vi "test8-LocalExternalStateRegistration.vi"(8 "error in (no error)":errorcluster, 11 "TestCase in":refnum<class "testcase-CSMBroadcast.lvclass">) -> (0 "error out":errorcluster, 3 "TestCase out":refnum<class "testcase-CSMBroadcast.lvclass">)   [LabVIEW 2017, in "testcase-CSMBroadcast.lvclass"]
uses:
  testcase-CSMBroadcast.lvclass
  0b17d103-e67b-41be-a9eb-a2ee1311ff1f.vi
  5999693e-4f8a-4b34-ae87-f34dff5771be.vi
  52a2a10a-a04b-4bad-8df4-e1eb944f47cc.vi
  826f03dd-b4b5-4c6b-9085-8edf6da4f43b.vi
  src/user.lib/_NEVSTOP/Communicable State Machine(CSM)/AdvanceAPI/CSM - Revert Arguments-Safe String.vi
  src/user.lib/_NEVSTOP/Communicable State Machine(CSM)/_Shared/Trim Single-line Text.vi
  src/user.lib/_NEVSTOP/Communicable State Machine(CSM)/AdvanceAPI/CSM - Make String Arguments Safe.vi
  src/user.lib/_NEVSTOP/Communicable State Machine(CSM)/AdvanceAPI/CSM - Break Down Multiple States String.vi
  src/user.lib/_NEVSTOP/Communicable State Machine(CSM)/AdvanceAPI/CSM - Keywords.vi
  src/user.lib/_NEVSTOP/Communicable State Machine(CSM)/_Polymophic/CSM - Replace Marks in Messages.vi
  src/user.lib/_NEVSTOP/Communicable State Machine(CSM)/AdvanceAPI/CSM - Get Module Attribute.vi
  <vilib>/addons/_JKI Toolkits/VI Tester/TestCase.llb/TestCase.lvclass
  src/user.lib/_NEVSTOP/Communicable State Machine(CSM)/Communicable State Machine.lvlib
  C:/Program Files (x86)/National Instruments/LabVIEW 2017/vi.lib/addons/_JKI Toolkits/VI Tester/TestCase.llb/TestCase.lvclass
panel:
  out "One-Shot Unregistrations":string
  out "One-Shot Registrations":string
  out "LoopCount 2":i32
  out "State History":string
  out "LoopCount":i32
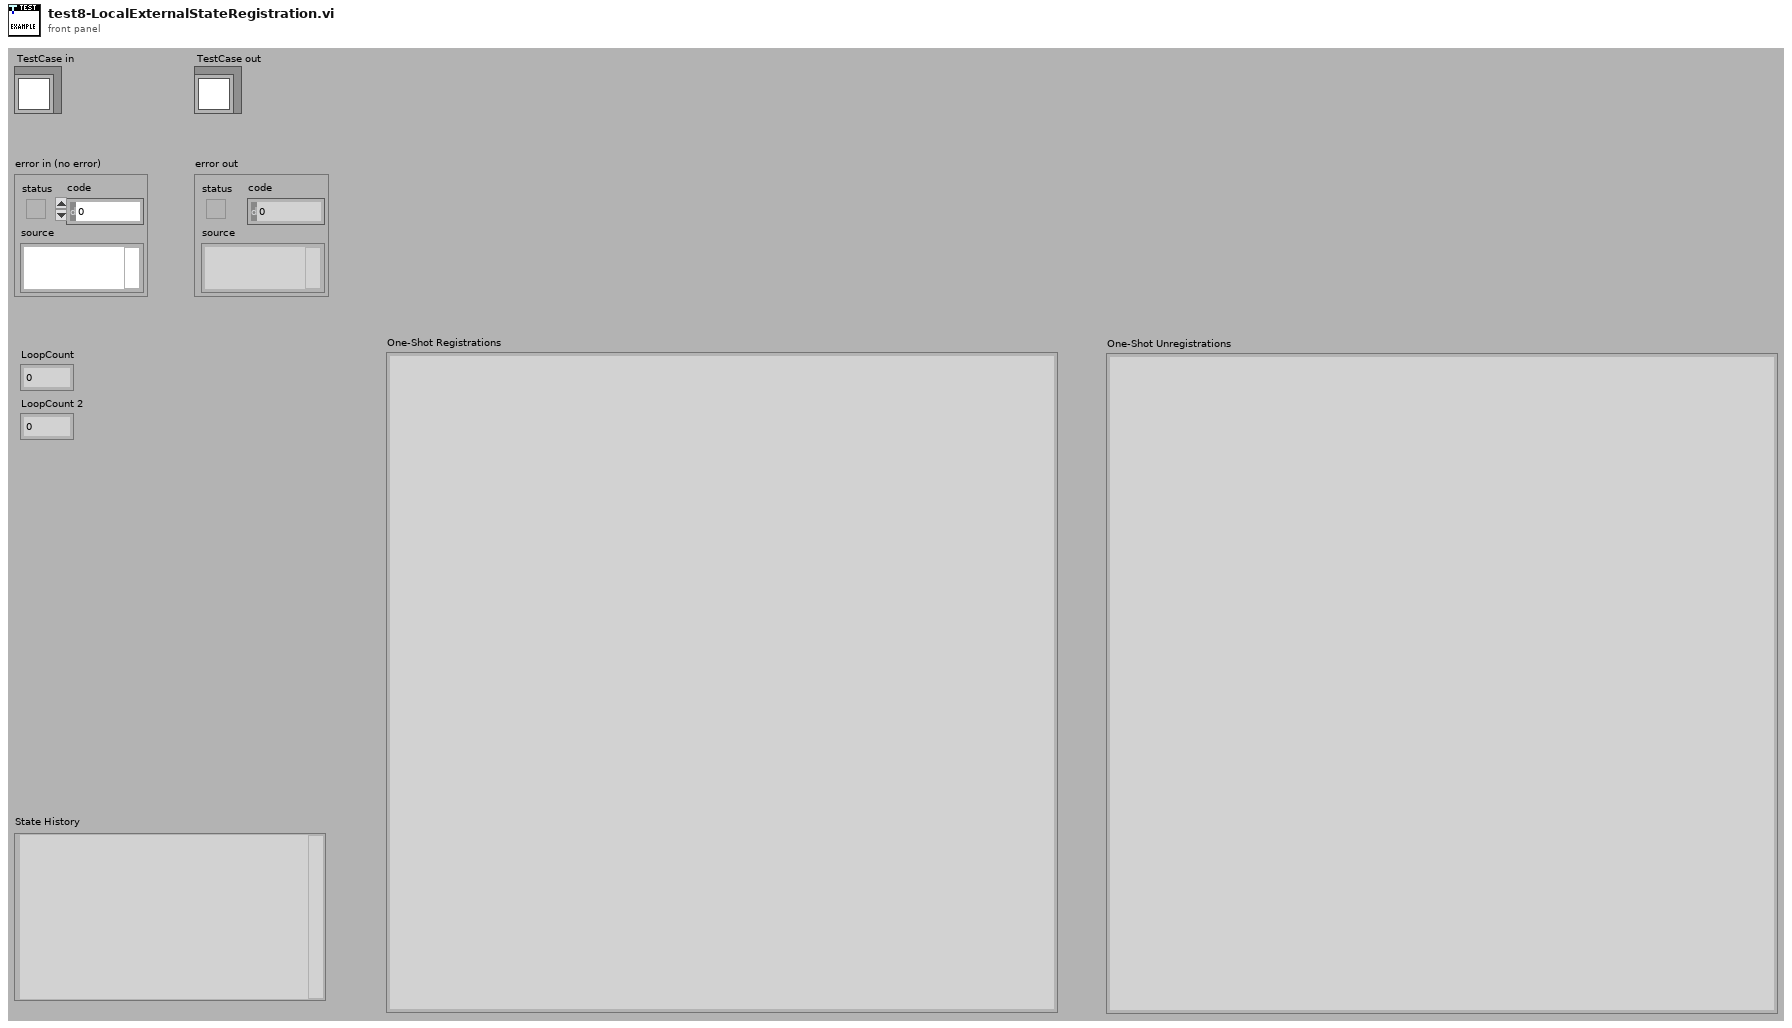
[diagram p1: front panel]
types:
  T1 = enum32{"Invalid", "Standard", "Closed", "Hidden", "Minimized", "Maximized"}
  T2 = enum32{"invalid app kind", "Development System", "Run Time System", "Student Edition", "Embedded LabVIEW", "Evaluation", "Custom"}
  T3 = typedef "Communicable State Machine.lvlib/_CSM_Response Source Message.ctl" = cluster{"‘State":string, "’Arguments":string, "’Error":errorcluster}
  T4 = cluster{"Current VI Reference":refnum<vi>, "Close Panel on Exit?":bool}
  T5 = cluster{"Core":cluster{"Current VI Reference":refnum<vi>, "Close Panel on Exit?":bool}, "Your Boolean data":bool, "Your string data":string}
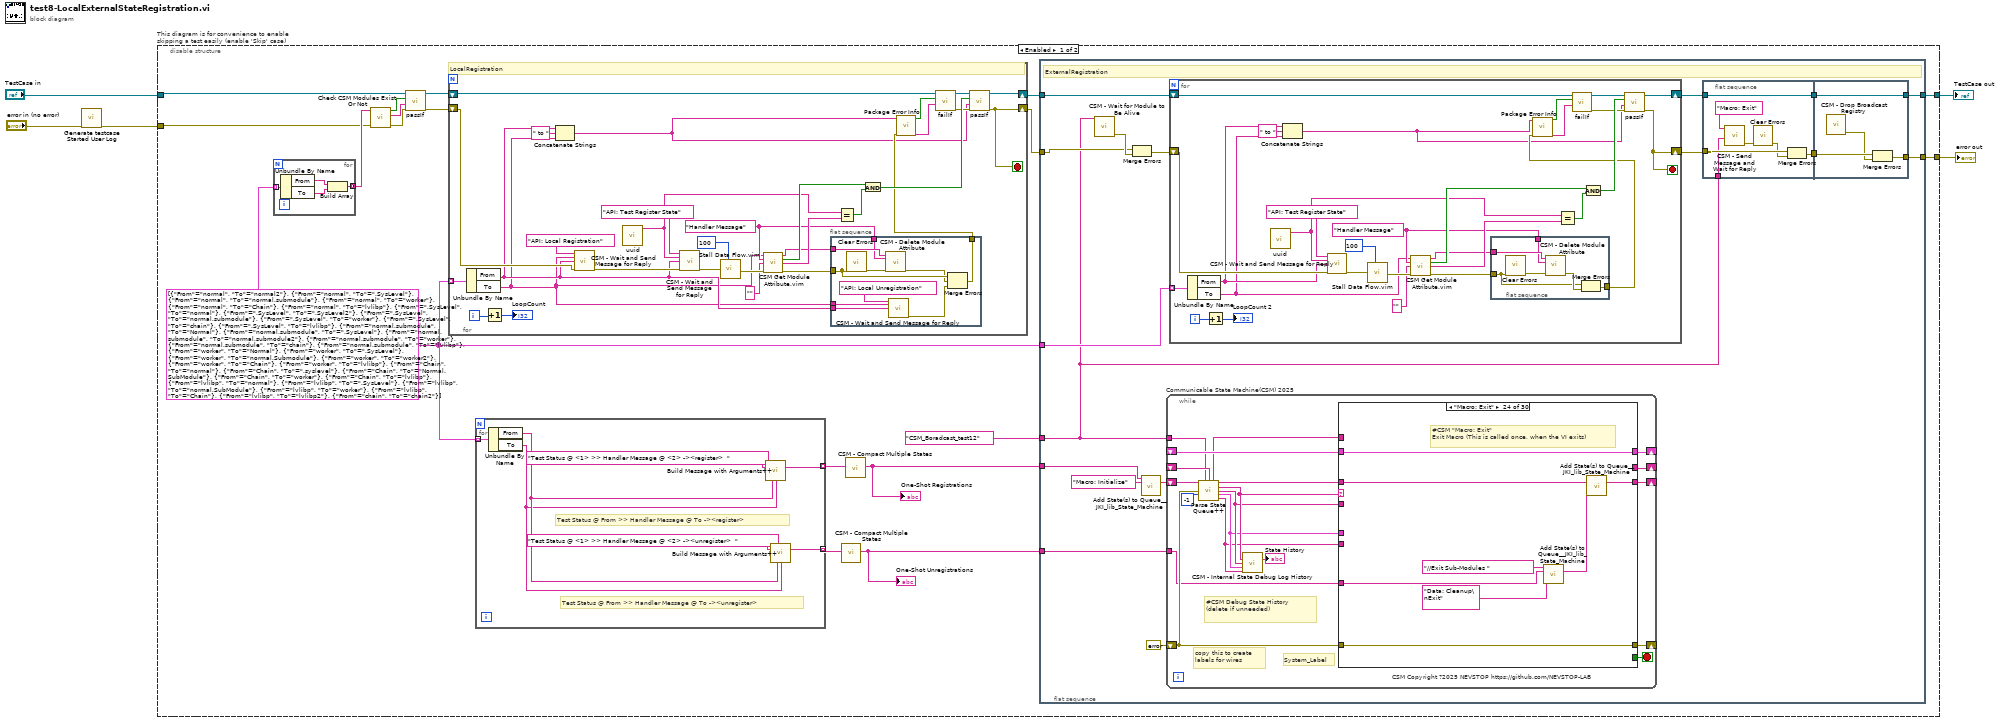
[diagram p0: block diagram]
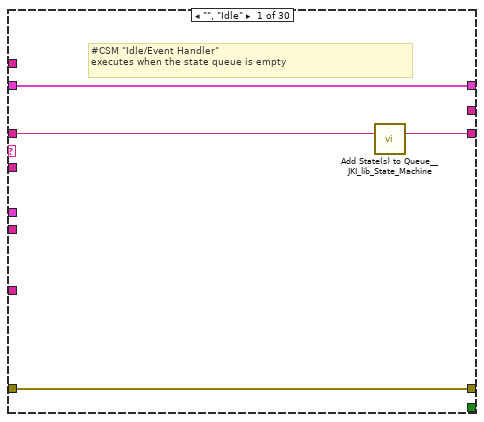
[diagram p2: hidden frame]
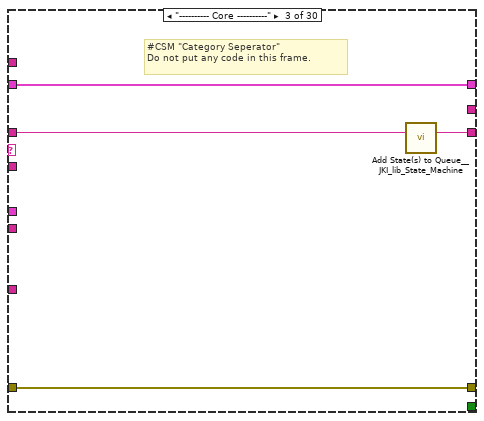
[diagram p4: hidden frame]
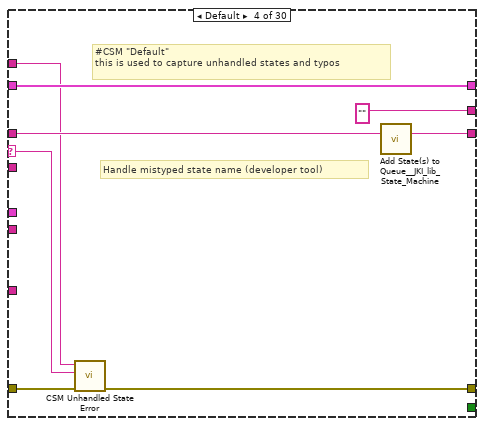
[diagram p5: hidden frame]
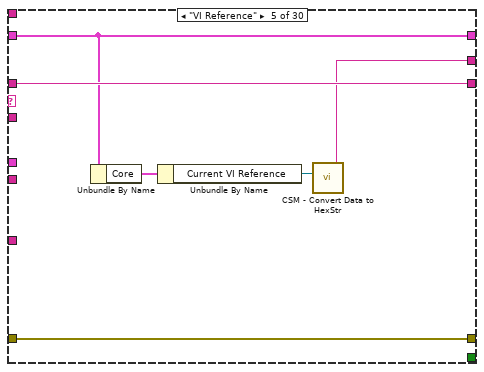
[diagram p6: hidden frame]
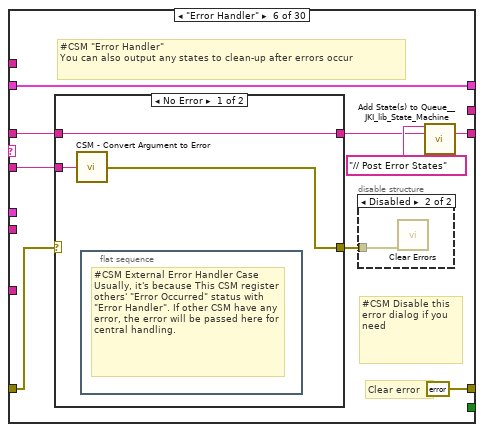
[diagram p7: hidden frame]
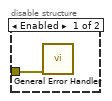
[diagram p8: hidden frame]
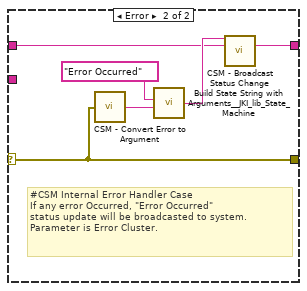
[diagram p9: hidden frame]
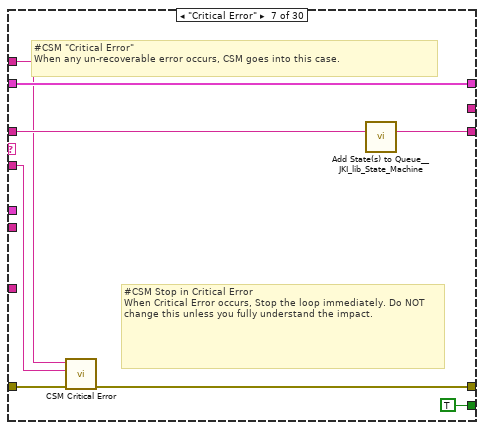
[diagram p10: hidden frame]
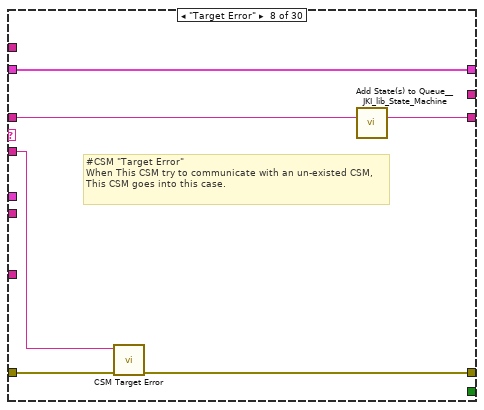
[diagram p11: hidden frame]
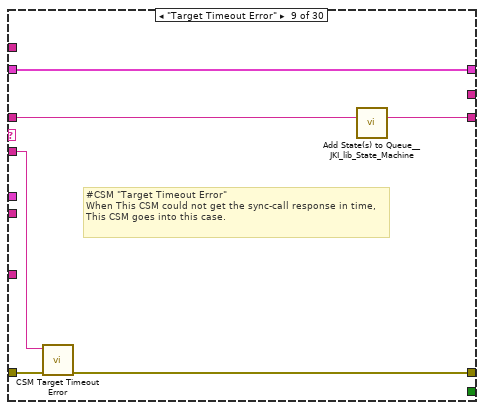
[diagram p12: hidden frame]
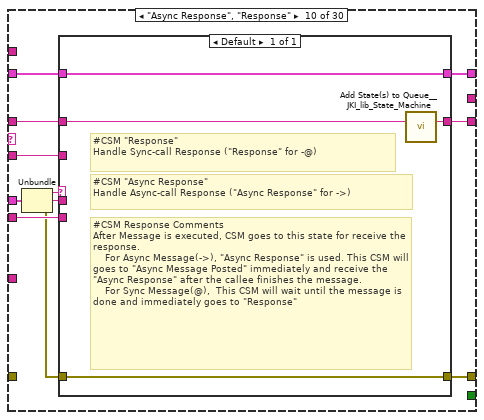
[diagram p13: hidden frame]
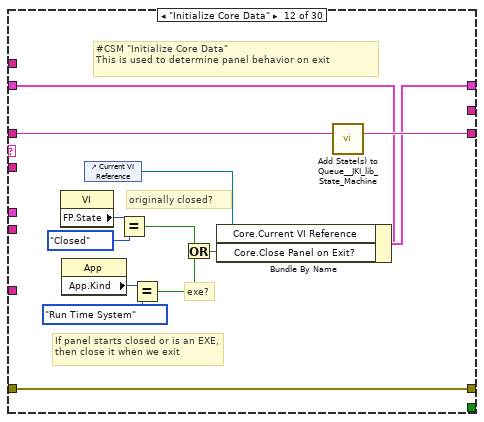
[diagram p15: hidden frame]
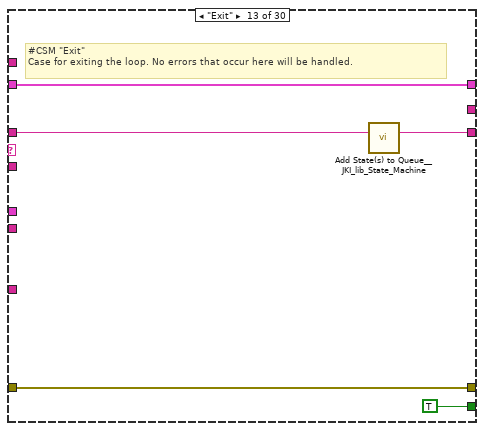
[diagram p16: hidden frame]
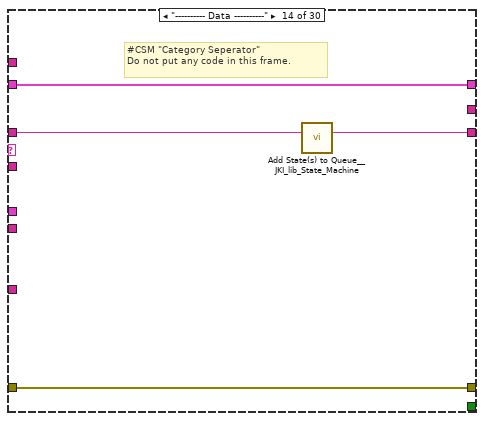
[diagram p17: hidden frame]
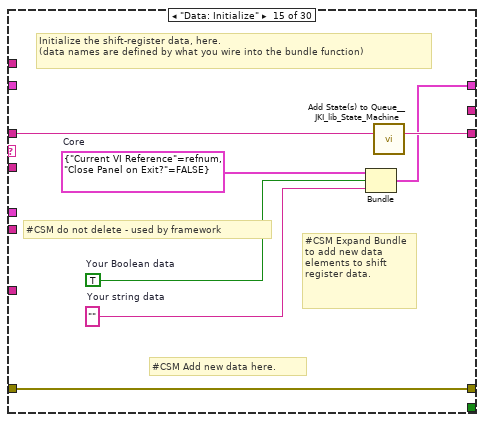
[diagram p18: hidden frame]
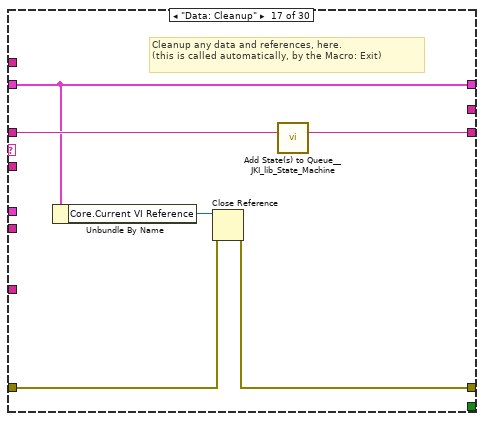
[diagram p20: hidden frame]
diagram:
  n1 = call "Generate testcase Started User Log.vi"("Error In"="error in (no error)") -> ("error out"=w1:errorcluster)  [unwired: 10 in]
  n2 = disable-structure "This diagram is for convenience to enable skipping a test easily (enable 'Skip' case)" shown="Enabled" {
    disable-tunnel: "TestCase in" -> [w11 w419]
    disable-tunnel: [w7 w417] -> w2
    disable-tunnel: [w17 w418] -> w4
    disable-tunnel: w1 -> [w8 w416]
    frame Enabled {
      w12 = cluster{"From":string, "To":string}[] [{"From"="normal", "To"="normal2"}, {"From"="normal", "To"=".SysLevel"}, {"From"="normal", "To"="normal.submodule"}, {"From"="normal", "To"="worker"}, {"From"="normal", "To"="Chain"}, {"From"="normal", "To"="lvlibp"}, {"From"=".SysLevel", "To"="normal"}, {"From"=".SysLevel", "To"=".SysLevel2"}, {"From"=".SysLevel", "To"="normal.submodule"}, {"From"=".SysLevel", "To"="worker"}, {"From"=".SysLevel", "To"="chain"}, {"From"=".SysLevel", "To"="lvlibp"}, {"From"="normal.submodule", "To"="Normal"}, {"From"="normal.submodule", "To"=".SysLevel"}, {"From"="normal.submodule", "To"="normal.submodule2"}, {"From"="normal.submodule", "To"="worker"}, {"From"="normal.submodule", "To"="chain"}, {"From"="normal.submodule", "To"="lvlibp"}, {"From"="worker", "To"="Normal"}, {"From"="worker", "To"=".SysLevel"}, {"From"="worker", "To"="normal.Submodule"}, {"From"="worker", "To"="worker2"}, {"From"="worker", "To"="Chain"}, {"From"="worker", "To"="lvlibp"}, {"From"="Chain", "To"="normal"}, {"From"="Chain", "To"=".syslevel"}, {"From"="Chain", "To"="Normal.SubModule"}, {"From"="Chain", "To"="worker"}, {"From"="Chain", "To"="lvlibp"}, {"From"="lvlibp", "To"="normal"}, {"From"="lvlibp", "To"=".SysLevel"}, {"From"="lvlibp", "To"="normal.SubModule"}, {"From"="lvlibp", "To"="worker"}, {"From"="lvlibp", "To"="Chain"}, {"From"="lvlibp", "To"="lvlibp2"}, {"From"="chain", "To"="chain2"}]
      n3 = for {
        tunnel: w12 -> [w27] mode=indexing
        tunnel: [w24] -> w15 mode=concatenating
        n4 = Unbundle By Name(w27) -> ("From"=w26:string, "To"=w25:string)
        n5 = Build Array(w26, w25) -> (w24:string[])
      }
      n6 = call "Check CSM Modules Exist Or Not.vi"("error in"=w8, "CSM names in"=w15) -> ("error out"=w13:errorcluster, "Debug string"=w14:string, "All Modules Exist?"=w16:bool)  [unwired: 7 in]
      n7 = call-dynamic "passIf.vi"("error in (no error)"=w13, "message (\"\")"=w14, "pass"=w16, "TestCase in"=w11) -> ("error out"=w9:errorcluster, "TestCase out"=w10:refnum<class "testcase-CSMBroadcast.lvclass">)  [unwired: 6 in]
      n8 = for {
        shift-right: [w38] -> w22
        shift-left: w9 -> [w39]
        shift-right: [w45] -> w23
        shift-left: w10 -> [w35]
        tunnel: w12 -> [w56] mode=indexing
        i -> [w58]
        stop <- w38 stop-if-true
        w40 = "Handler Message" ("To")
        # "LocalRegistration"
        n9 = Unbundle By Name(w56) -> ("From"=w31:string, "To"=w30:string)
        n10 = Increment(x=w58) -> (x+1=→"LoopCount":i32)
        n11 = Concatenate Strings(w31, " to " ("string"), w30) -> (w28:string)
        n12 = call "CSM - Wait and Send Message for Reply.vi"("State"="API: Local Registration", "Arguments (\"\")"=w30, "Target Module"=w31, "Error In (No Error)"=w39) -> ("error out"=w53:errorcluster)  [unwired: 8 in, 3 out]
        n13 = call "uuid.vi"() -> ("UUID"=w47:string)  [unwired: 11 in]
        n14 = call "CSM - Wait and Send Message for Reply.vi"("State"="API: Test Register State", "Arguments (\"\")"=w47, "Target Module"=w31, "Error In (No Error)"=w53) -> ("error out"=w52:errorcluster)  [unwired: 8 in, 3 out]
        n15 = call "Stall Data Flow.vim"("value in"=w52, "milliseconds to wait"=u32 100) -> ("value out"=w50:errorcluster)  [unwired: 1 out]
        n16 = call "CSM Get Module Attribute.vim"("CSM Name"=w30, "Attribute"=w40, "Default Value (Empty Variant)"="", "Error In"=w50) -> ("CSM Name (Dup)"=w41:string, "Found"=w49:bool, "Value"=w46:string, "error out"=w42:errorcluster)  [unwired: 7 in, 1 out]
        n17 = flat-sequence {
          tunnel: w42 -> [w62]
          tunnel: w41 -> [w67]
          tunnel: w40 -> [w66]
          tunnel: w30 -> [w64]
          tunnel: w31 -> [w63]
          tunnel: [w59] -> w32
          frame #0 {
            n18 = call <vilib>:"Clear Errors.vi"("error in (no error)"=w62) -> ("error out"=w68:errorcluster)  [unwired: 5 in, 1 out]
            n19 = call "CSM - Delete Module Attribute.vi"("CSM Name"=w67, "Attribute"=w66, "Error In"=w68) -> ("error out"=w61:errorcluster)  [unwired: 9 in, 3 out]
            n20 = call "CSM - Wait and Send Message for Reply.vi"("State"="API: Local Unregistration", "Arguments (\"\")"=w64, "Target Module"=w63) -> ("error out"=w60:errorcluster)  [unwired: 9 in, 3 out]
            n21 = Merge Errors(w62, w61, w60) -> (w59:errorcluster)
          }
        }
        n22 = Equal?(x=w47, y=w46) -> (x = y?=w44:bool)
        n23 = And(x=w49, y=w44) -> (x .and. y?=w43:bool)
        n24 = call "Package Error Info.vi"("error in"=w32, "String in"=w28) -> ("packed error info out"=w36:string, "error status"=w37:bool)  [unwired: 8 in]
        n25 = call-dynamic "failIf.vi"("message (\"\")"=w36, "fail"=w37, "TestCase in"=w35) -> ("error out"=w33:errorcluster, "TestCase out"=w34:refnum<class "testcase-CSMBroadcast.lvclass">)  [unwired: 7 in]
        n26 = call-dynamic "passIf.vi"("error in (no error)"=w33, "message (\"\")"=w28, "pass"=w43, "TestCase in"=w34) -> ("error out"=w38:errorcluster, "TestCase out"=w45:refnum<class "testcase-CSMBroadcast.lvclass">)  [unwired: 6 in]
      }
      n27 = for {
        tunnel: w12 -> [w74] mode=indexing
        tunnel: [w73] -> w21 mode=indexing
        tunnel: [w69] -> w19 mode=indexing
        # "Test Status @ From >> Handler Message @ To -><unregister>"
        # "Test Status @ From >> Handler Message @ To -><register>"
        n28 = Unbundle By Name(w74) -> ("From"=w71:string, "To"=w70:string)
        n29 = call-poly "Build Message with Arguments++.vi"("States With Replace Token"="Test Status @ <1> >> Handler Message @ <2> -><register>  " ("State"), "<1>"=w71, "<2>"=w70) -> ("States"=w73:string)  [unwired: 12 in]
        n30 = call-poly "Build Message with Arguments++.vi"("States With Replace Token"="Test Status @ <1> >> Handler Message @ <2> -><unregister>  " ("State"), "<1>"=w71, "<2>"=w70) -> ("States"=w69:string)  [unwired: 12 in]
      }
      n31 = call "CSM - Compact Multiple States.vi"("Multiple States"=w19) -> ("States"=w18:string)  [unwired: 9 in]
      "One-Shot Unregistrations" <- w18
      n32 = call "CSM - Compact Multiple States.vi"("Multiple States"=w21) -> ("States"=w20:string)  [unwired: 9 in]
      "One-Shot Registrations" <- w20
      n33 = flat-sequence {
        tunnel: w23 -> [w89]
        tunnel: w22 -> [w83]
        tunnel: w12 -> [w88]
        tunnel: w20 -> [w86]
        tunnel: w18 -> [w82]
        tunnel: [w80] -> w17
        tunnel: [w77] -> w7
        tunnel: "CSM_Boradcast_test12" ("Name (\"\" to Use UUID)") -> [w76]
        frame #0 {
          # "ExternalRegistration"
          n34 = call "CSM - Wait for Module to Be Alive.vi"("CSM Name"=w76) -> ("error out"=w87:errorcluster)  [unwired: 12 in, 2 out]
          n35 = Merge Errors(w83, w87) -> (w84:errorcluster)
          n36 = call <vilib>:"Add State(s) to Queue__JKI_lib_State_Machine.vi"("State(s) in Front (\"\")"=w86, "State(s) in (\"\")"="Macro: Initialize" ("Init State(\"Macro: Initialize\")")) -> ("States Out"=w90:string)  [unwired: 13 in]
          n37 = while "Communicable State Machine(CSM) 2025" {
            shift-right: [w152] -> _
            shift-left: _ -> [w151]
            shift-right: [w155] -> _
            shift-left: errorcluster {"status"=FALSE, "code"=0, "source"=""} ("error out") -> [w150]
            shift-right: [w154] -> _
            shift-left: w90 -> [w156]
            shift-right: [w149] -> _
            shift-left: _ -> [w143]
            tunnel: w82 -> [w140]
            tunnel: w76 -> [w139]
            stop <- w153 stop-if-true
            # "#CSM Debug State History\n(delete if unneeded)"
            # "copy this to create labels for wires"
            # "System_Label"
            # "CSM Copyright ?2025 NEVSTOP https://github.com/NEVSTOP-LAB"
            n38 = call "Parse State Queue++.vi"("State Queue"=w156, "Name (\"\" to Use UUID)"=w139, "Response Arguments"=w143, "Previous Error"=w150, "Dequeue (1 ms)"=-1 ("Timeout")) -> ("Name Used"=w144:string, "Remaining States"=w157:string, "Current State"=w148:string, "Arguments"=w147:string, "Additional Information"=w146:T3, "Source CSM"=w145:string)  [unwired: 5 in]
            n39 = call "CSM - Internal State Debug Log History.vi"("State"=w148, "Arguments (\"\")"=w147, ">> Response Source Message >>"=w146, "Source (\"\")"=w145) -> ("Debug Log"=→"State History":string)  [unwired: 11 in]
            n40 = case shown="\"Macro: Exit\"" w148 {
              selector: w148 -> [_ _ _ w171 _ _ _ _ _ _ _ _ _ _ _ _ _ _ _ _ _ _ _ _ _ _ _ _ _ _]
              tunnel: w157 -> [w158 w163 w168 w175 w181 w187 w208 w214 w220 w228 w239 w253 w258 w262 w269 w271 w278 w282 w286 w292 w307 w376 w381 w389 w391 w395 w400 w407 w411 w415]
              tunnel: w147 -> [_ _ _ _ _ w186 w204 w213 w218 w227 _ _ _ _ _ _ _ _ _ w287 w301 _ _ _ _ _ w398 _ _ _]
              tunnel: w151 -> [w159 w162 w165 w173 w180 w190 w209 w215 w221 w230 w238 w246 w256 w259 _ w270 w273 w279 w284 w290 w303 w373 w378 w386 w390 w394 w399 w404 w408 w412]
              tunnel: [w160 w164 w166 w169 w182 errorcluster {"status"=FALSE, "code"=0, "source"=""} ("error out") w205 w211 w217 w233 w240 w250 w255 w260 w266 w272 w274 w280 w283 w288 w304 w374 w379 w387 w392 w396 w401 w405 w409 w413] -> w155
              tunnel: w150 -> [w160 w164 w166 w176 w182 w188 w210 w212 w219 _ w240 w250 w255 w260 w266 w272 w275 w280 w283 w289 w305 w374 w379 w387 w392 w396 w401 w405 w409 w413]
              tunnel: [w161 w163 w167 w174 w181 w183 w207 w216 w222 w229 w239 w252 w257 w261 w268 w271 w277 w281 w285 w291 w306 w375 w380 w388 w391 w395 w400 w406 w410 w414] -> w154
              tunnel: [_ _ _ _ _ _ TRUE _ _ _ _ _ TRUE _ _ _ _ _ _ _ _ _ _ _ _ _ _ _ _ _] -> w153
              tunnel: [w159 w162 w165 w173 w180 w190 w209 w215 w221 w231 w238 w251 w256 w259 w267 w270 w273 w279 w284 w290 w303 w373 w378 w386 w390 w394 w399 w404 w408 w412] -> w152
              tunnel: w145 -> [_ _ _ _ _ _ _ _ _ w225 _ _ _ _ _ _ _ _ _ _ _ _ _ _ _ _ _ _ _ _]
              tunnel: w146 -> [_ _ _ _ _ _ _ _ _ w232 _ _ _ _ _ _ _ _ _ _ _ _ _ _ _ _ _ _ _ _]
              tunnel: [_ _ _ "" w177 _ _ _ _ _ _ _ _ _ _ _ _ _ _ _ _ _ _ _ _ "API1 Response" w397 _ _ _] -> w149
              tunnel: w144 -> [_ _ _ w170 _ _ w203 _ _ _ _ _ _ _ _ _ _ _ _ _ _ _ _ _ _ _ _ _ _ _]
              tunnel: w140 -> [_ _ _ _ _ _ _ _ _ _ _ _ _ _ _ _ _ _ _ _ _ _ _ w382 _ _ _ _ _ _]
              frame "", "Idle" {
                # "#CSM \"Idle/Event Handler\"\nexecutes when the state queue is empty"
                n41 = call <vilib>:"Add State(s) to Queue__JKI_lib_State_Machine.vi"("State(s) in (\"\")"=w158) -> ("States Out"=w161:string)  [unwired: 14 in]
              }
              frame "CSM Documentation" {
                # "#CSM README FIRST\n\nCommunicable State Machine(CSM) is a LabVIEW application framework that builds upon JKI State Machine(JKISM). It follows the pattern of JKISM and extends the keywords to describe message communication between modules, including concepts such as Sync-Message, Async-Message, Subscription/Unsubscription of status - essential elements for creating reusable code modules. For more information, please visit the CSM wiki: https://nevstop-lab.github.io/CSM-Wiki/\n\nFor instructions on JKI State Machine, visit: http://jki.net/state-machine/\nFor information about CSM, visit: https://github.com/NEVSTOP-LAB"
                # "#CSM \"Documentation\"\nCase for holding CSM Documenation"
              }
              frame "---------- Core ----------" {
                # "#CSM \"Category Seperator\"\nDo not put any code in this frame."
                n42 = call <vilib>:"Add State(s) to Queue__JKI_lib_State_Machine.vi"("State(s) in (\"\")"=w168) -> ("States Out"=w167:string)  [unwired: 14 in]
              }
              frame Default {
                # "#CSM \"Default\"\nthis is used to capture unhandled states and typos"
                # "Handle mistyped state name (developer tool)"
                n43 = call "CSM Unhandled State Error.vi"("error in (no error)"=w176, "Undefined State"=w171, "CSM Name"=w170) -> ("error out"=w169:errorcluster)  [unwired: 8 in]
                n44 = call <vilib>:"Add State(s) to Queue__JKI_lib_State_Machine.vi"("State(s) in (\"\")"=w175) -> ("States Out"=w174:string)  [unwired: 14 in]
              }
              frame "VI Reference" {
                n45 = Unbundle By Name(w180) -> ("Core"=w179:T4)
                n46 = Unbundle By Name(w179) -> ("Current VI Reference"=w178:refnum<vi>)
                n47 = call "CSM - Convert Data to HexStr.vi"("Variant"=w178) -> ("HEX String (0-9,A-F)"=w177:string)  [unwired: 8 in]
              }
              frame "Error Handler" {
                # "#CSM Disable this error dialog if you need"
                # "#CSM \"Error Handler\"\nYou can also output any states to clean-up after errors occur"
                # "Clear error"
                n48 = case shown="No Error" w188 {
                  selector: w188 -> [_ w197]
                  tunnel: [w196 w199] -> w184
                  tunnel: w187 -> [w196 w198]
                  tunnel: w186 -> [w195 _]
                  tunnel: [w194 w197] -> w189
                  frame No Error {
                    n49 = call "CSM - Convert Argument to Error.vi"("Argument"=w195) -> ("Error"=w194:errorcluster)  [unwired: 4 in]
                    n50 = flat-sequence {
                      frame #0 {
                        # "#CSM External Error Handler Case\nUsually, it's because This CSM register others' \"Error Occurred\" status with \"Error Handler\". If other CSM have any error, the error will be passed here for central handling."
                      }
                    }
                  }
                  frame Error {
                    # "#CSM Internal Error Handler Case \nIf any error Occurred, \"Error Occurred\" \nstatus update will be broadcasted to system.\nParameter is Error Cluster."
                    n51 = call "CSM - Convert Error to Argument.vi"("Error"=w197) -> ("Argument"=w201:string)  [unwired: 4 in]
                    n52 = call <vilib>:"Build State String with Arguments__JKI_lib_State_Machine.vi"("Arguments (\"\")"=w201, "State"="Error Occurred" ("Status with Arguments")) -> ("State with Arguments"=w200:string)  [unwired: 4 in]
                    n53 = call "CSM - Broadcast Status Change.vi"("Status With Arguments"=w200, "State Queue"=w198) -> ("Remaining States"=w199:string)  [unwired: 13 in]
                  }
                }
                n54 = disable-structure shown="Disabled" {
                  disable-tunnel: w189 -> [w192 w193]
                  frame Enabled {
                    n55 = call <vilib>:"General Error Handler.vi"("error in (no error)"=w192) -> ()  [unwired: 10 in, 5 out]
                  }
                  frame Disabled {
                    n56 = call <vilib>:"Clear Errors.vi"("error in (no error)"=w193) -> ()  [unwired: 5 in, 2 out]
                  }
                }
                n57 = call <vilib>:"Add State(s) to Queue__JKI_lib_State_Machine.vi"("State(s) in Front (\"\")"="// Post Error States", "State(s) in (\"\")"=w184) -> ("States Out"=w183:string)  [unwired: 13 in]
              }
              frame "Critical Error" {
                # "#CSM Stop in Critical Error\nWhen Critical Error occurs, Stop the loop immediately. Do NOT change this unless you fully understand the impact."
                # "#CSM \"Critical Error\"\nWhen any un-recoverable error occurs, CSM goes into this case."
                n58 = call "CSM Critical Error.vi"("error in (no error)"=w210, "Arugments (As Reason)"=w204, "CSM Name"=w203) -> ("error out"=w205:errorcluster)  [unwired: 8 in]
                n59 = call <vilib>:"Add State(s) to Queue__JKI_lib_State_Machine.vi"("State(s) in (\"\")"=w208) -> ("States Out"=w207:string)  [unwired: 14 in]
              }
              frame "Target Error" {
                # "#CSM \"Target Error\"\nWhen This CSM try to communicate with an un-existed CSM, This CSM goes into this case."
                n60 = call "CSM Target Error.vi"("error in (no error)"=w212, "Arguments (As CSM Name)"=w213) -> ("error out"=w211:errorcluster)  [unwired: 9 in]
                n61 = call <vilib>:"Add State(s) to Queue__JKI_lib_State_Machine.vi"("State(s) in (\"\")"=w214) -> ("States Out"=w216:string)  [unwired: 14 in]
              }
              frame "Target Timeout Error" {
                # "#CSM \"Target Timeout Error\"\nWhen This CSM could not get the sync-call response in time, This CSM goes into this case."
                n62 = call "CSM Target Timeout Error.vi"("error in (no error)"=w219, "Arguments (As CSM Name)"=w218) -> ("error out"=w217:errorcluster)  [unwired: 9 in]
                n63 = call <vilib>:"Add State(s) to Queue__JKI_lib_State_Machine.vi"("State(s) in (\"\")"=w220) -> ("States Out"=w222:string)  [unwired: 14 in]
              }
              frame "Async Response", "Response" {
                n64 = Unbundle(w232) -> ("‘State"=w226:string, "’Arguments"=w224:string, "’Error"=w223:errorcluster)
                n65 = case shown="Default" w226 {
                  tunnel: [w237] -> w233
                  tunnel: w223 -> [w237]
                  tunnel: [w236] -> w231
                  tunnel: w230 -> [w236]
                  tunnel: [w234] -> w229
                  tunnel: w228 -> [w235]
                  tunnel: w227 -> [_]
                  tunnel: w225 -> [_]
                  tunnel: w224 -> [_]
                  frame Default {
                    # "#CSM Response Comments\nAfter Message is executed, CSM goes to this state for receive the response.\n    For Async Message(->), \"Async Response\" is used. This CSM will goes to \"Async Message Posted\" immediately and receive the \"Async Response\" after the callee finishes the message.\n    For Sync Message(@),  This CSM will wait until the message is done and immediately goes to \"Response\""
                    # "#CSM \"Async Response\"\nHandle Async-call Response (\"Async Response\" for ->)"
                    # "#CSM \"Response\"\nHandle Sync-call Response (\"Response\" for -@)"
                    n66 = call <vilib>:"Add State(s) to Queue__JKI_lib_State_Machine.vi"("State(s) in (\"\")"=w235) -> ("States Out"=w234:string)  [unwired: 14 in]
                  }
                }
              }
              frame "Async Message Posted" {
                # "#CSM \"Async Message Posted\"\nAfter Async Message is posted (-> or ->| ), CSM goes to this state for post-action.\nYou can use Argument - State to tell which Async Message is called."
              }
              frame "Initialize Core Data" {
                # "#CSM \"Initialize Core Data\"\nThis is used to determine panel behavior on exit"
                # "originally closed?"
                # "exe?"
                # "If panel starts closed or is an EXE, then close it when we exit"
                n67 = property class="VI"() -> ("FP.State"=w243:T1)  [unwired: 2 in, 2 out]
                n68 = property class="App"() -> ("App.Kind"=w249:T2)  [unwired: 2 in, 2 out]
                n69 = control-ref of="Current VI Reference"() -> (w244:refnum<vi>)
                n70 = Equal?(x=w243, y=T1."Closed" ("Front Panel Window:State")) -> (x = y?=w241:bool)
                n71 = Equal?(x=w249, y=T2."Run Time System" ("Application:Kind")) -> (x = y?=w247:bool)
                n72 = Or(x=w241, y=w247) -> (x .or. y?=w245:bool)
                n73 = Bundle By Name(cluster=w246, "Core.Current VI Reference"=w244, "Core.Close Panel on Exit?"=w245) -> (w251:T5)
                n74 = call <vilib>:"Add State(s) to Queue__JKI_lib_State_Machine.vi"("State(s) in (\"\")"=w253) -> ("States Out"=w252:string)  [unwired: 14 in]
              }
              frame "Exit" {
                # "#CSM \"Exit\"\nCase for exiting the loop. No errors that occur here will be handled."
                n75 = call <vilib>:"Add State(s) to Queue__JKI_lib_State_Machine.vi"("State(s) in (\"\")"=w258) -> ("States Out"=w257:string)  [unwired: 14 in]
              }
              frame "---------- Data ----------" {
                # "#CSM \"Category Seperator\"\nDo not put any code in this frame."
                n76 = call <vilib>:"Add State(s) to Queue__JKI_lib_State_Machine.vi"("State(s) in (\"\")"=w262) -> ("States Out"=w261:string)  [unwired: 14 in]
              }
              frame "Data: Initialize" {
                w263 = T4 {"Current VI Reference"=refnum, "Close Panel on Exit?"=FALSE}  # Core
                w265 = TRUE  # Your Boolean data
                w264 = ""  # Your string data
                # "#CSM do not delete - used by framework"
                # "#CSM Expand Bundle to add new data elements to shift register data."
                # "#CSM Add new data here."
                # "Initialize the shift-register data, here.\n(data names are defined by what you wire into the bundle function)"
                n77 = Bundle("Core"=w263, "Your Boolean data"=w265, "Your string data"=w264) -> (w267:T5)  [unwired: 1 in]
                n78 = call <vilib>:"Add State(s) to Queue__JKI_lib_State_Machine.vi"("State(s) in (\"\")"=w269) -> ("States Out"=w268:string)  [unwired: 14 in]
              }
              frame "Data: Update Indicators" {
              }
              frame "Data: Cleanup" {
                # "Cleanup any data and references, here.\n(this is called automatically, by the Macro: Exit)"
                n79 = Unbundle By Name(w273) -> ("Core.Current VI Reference"=w276:refnum<vi>)
                n80 = Close Reference(reference=w276, error in (no error)=w275) -> (error out=w274:errorcluster)
                n81 = call <vilib>:"Add State(s) to Queue__JKI_lib_State_Machine.vi"("State(s) in (\"\")"=w278) -> ("States Out"=w277:string)  [unwired: 14 in]
              }
              frame "---------- UI ----------" {
                # "#CSM \"Category Seperator\"\nDo not put any code in this frame."
                n82 = call <vilib>:"Add State(s) to Queue__JKI_lib_State_Machine.vi"("State(s) in (\"\")"=w282) -> ("States Out"=w281:string)  [unwired: 14 in]
              }
              frame "UI: Initialize" {
                # "#CSM \"UI: Initialize\"\nInitialize the User Interface, here.\n(this is called automatically, by the Macro: Init)"
                n83 = call <vilib>:"Add State(s) to Queue__JKI_lib_State_Machine.vi"("State(s) in (\"\")"=w286) -> ("States Out"=w285:string)  [unwired: 14 in]
              }
              frame "UI: Cursor Set" {
                # "#CSM \"UI: Cursor Set\"\nSet and Unset Cursor Busy.\n(Usage: \"UI: Cursor Set >> Busy|Idle\")"
                # "Argument"
                n84 = disable-structure shown="TARGET_TYPE!=Windows" {
                  disable-tunnel: w289 -> [w295 w300]
                  disable-tunnel: [w294 w300] -> w288
                  disable-tunnel: w287 -> [w293 _]
                  frame condition #0 (active) {
                    n85 = case shown="\"Idle\", Default" w293 {
                      tunnel: w295 -> [w297 w299]
                      tunnel: [w296 w298] -> w294
                      frame "Idle", Default {
                        n86 = call <vilib>:"Unset Busy.vi"("error in (no error)"=w297) -> ("error out"=w296:errorcluster)  [unwired: 10 in]
                      }
                      frame "Busy" {
                        n87 = call <vilib>:"Set Busy.vi"("error in (no error)"=w299) -> ("error out"=w298:errorcluster)  [unwired: 9 in, 1 out]
                      }
                    }
                  }
                  frame condition #1 {
                  }
                }
                n88 = call <vilib>:"Add State(s) to Queue__JKI_lib_State_Machine.vi"("State(s) in (\"\")"=w292) -> ("States Out"=w291:string)  [unwired: 14 in]
              }
              frame "UI: Front Panel State" {
                # "#CSM \"UI: Front Panel State\"\nSet Front Panel Open or Closed\n(Usage: \"UI: Front Panel State >> Open|Close\")"
                # "Argument"
                n89 = Unbundle By Name(w303) -> ("Core.Current VI Reference"=w302:refnum<vi>)
                n90 = call <vilib>:"Add State(s) to Queue__JKI_lib_State_Machine.vi"("State(s) in (\"\")"=w307) -> ("States Out"=w306:string)  [unwired: 14 in]
                n91 = case shown="\"Close\", \"Closed\"" w301 {
                  tunnel: w305 -> [w313 w328 w339 w352 w365]
                  tunnel: [w315 w329 w341 w354 w367] -> w304
                  tunnel: w302 -> [w314 w326 w340 w353 w366]
                  frame "Open", "Standard", Default {
                    w308 = T1."Standard" ("State")
                    n92 = property class="VI"(reference=w314, error in=w313) -> (reference out=w311:refnum<vi>, error out=w312:errorcluster, "FP.State"=w310:T1)
                    n93 = Not Equal?(x=w310, y=w308) -> (x != y?=w309:bool)
                    n94 = case shown="True" w309 {
                      tunnel: [w319 w321] -> w315
                      tunnel: w312 -> [w318 w321]
                      tunnel: w311 -> [w317 _]
                      tunnel: w308 -> [w316 _]
                      frame True {
                        n95 = invoke class="VI" method="FP.Open"(reference=w317, error in=w318, "Activate"=TRUE, "State"=w316) -> (error out=w319:errorcluster)  [unwired: 1 in, 4 out]
                      }
                      frame False {
                      }
                    }
                  }
                  frame "Close", "Closed" {
                    n96 = property class="VI"(reference=w326, error in=w328) -> (reference out=w325:refnum<vi>, error out=w327:errorcluster, "FP.State"=w323:T1)
                    n97 = Not Equal?(x=w323, y=T1."Closed" ("Front Panel Window:State")) -> (x != y?=w322:bool)
                    n98 = case shown="False" w322 {
                      tunnel: [w330 w333] -> w329
                      tunnel: w327 -> [w330 w332]
                      tunnel: w325 -> [_ w331]
                      frame False {
                      }
                      frame True {
                        n99 = invoke class="VI" method="FP.Close"(reference=w331, error in=w332) -> (error out=w333:errorcluster)  [unwired: 1 in, 2 out]
                      }
                    }
                  }
                  frame "Hidden", "Hide" {
                    w334 = T1."Hidden" ("State")
                    n100 = property class="VI"(reference=w340, error in=w339) -> (reference out=w337:refnum<vi>, error out=w338:errorcluster, "FP.State"=w336:T1)
                    n101 = Not Equal?(x=w336, y=w334) -> (x != y?=w335:bool)
                    n102 = case shown="True" w335 {
                      tunnel: [w345 w346] -> w341
                      tunnel: w338 -> [w344 w346]
                      tunnel: w337 -> [w343 _]
                      tunnel: w334 -> [w342 _]
                      frame True {
                        n103 = invoke class="VI" method="FP.Open"(reference=w343, error in=w344, "State"=w342) -> (error out=w345:errorcluster)  [unwired: 2 in, 4 out]
                      }
                      frame False {
                      }
                    }
                  }
                  frame "Minimize", "Minimized" {
                    w347 = T1."Minimized" ("State")
                    n104 = property class="VI"(reference=w353, error in=w352) -> (reference out=w350:refnum<vi>, error out=w351:errorcluster, "FP.State"=w349:T1)
                    n105 = Not Equal?(x=w349, y=w347) -> (x != y?=w348:bool)
                    n106 = case shown="True" w348 {
                      tunnel: [w358 w359] -> w354
                      tunnel: w351 -> [w357 w359]
                      tunnel: w350 -> [w356 _]
                      tunnel: w347 -> [w355 _]
                      frame True {
                        n107 = invoke class="VI" method="FP.Open"(reference=w356, error in=w357, "State"=w355) -> (error out=w358:errorcluster)  [unwired: 2 in, 4 out]
                      }
                      frame False {
                      }
                    }
                  }
                  frame "Maximize", "Maximized" {
                    w360 = T1."Maximized" ("State")
                    n108 = property class="VI"(reference=w366, error in=w365) -> (reference out=w363:refnum<vi>, error out=w364:errorcluster, "FP.State"=w362:T1)
                    n109 = Not Equal?(x=w362, y=w360) -> (x != y?=w361:bool)
                    n110 = case shown="True" w361 {
                      tunnel: [w371 w372] -> w367
                      tunnel: w364 -> [w370 w372]
                      tunnel: w363 -> [w369 _]
                      tunnel: w360 -> [w368 _]
                      frame True {
                        n111 = invoke class="VI" method="FP.Open"(reference=w369, error in=w370, "State"=w368) -> (error out=w371:errorcluster)  [unwired: 2 in, 4 out]
                      }
                      frame False {
                      }
                    }
                  }
                }
              }
              frame "---------- Macro ----------" {
                # "#CSM \"Category Seperator\"\nDo not put any code in this frame."
                n112 = call <vilib>:"Add State(s) to Queue__JKI_lib_State_Machine.vi"("State(s) in (\"\")"=w376) -> ("States Out"=w375:string)  [unwired: 14 in]
              }
              frame "Macro: Initialize" {
                # "#CSM \"Macro: Initialize\"\nInitialization Macro (This is called once, when the VI starts)"
                n113 = call <vilib>:"Add State(s) to Queue__JKI_lib_State_Machine.vi"("State(s) in Front (\"\")"="Data: Initialize\nInitialize Core Data\nData: Update Indicators", "State(s) in (\"\")"=w381) -> ("States Out"=w380:string)  [unwired: 13 in]
              }
              frame "Macro: Exit" {
                # "#CSM \"Macro: Exit\"\nExit Macro (This is called once, when the VI exits)"
                n114 = call <vilib>:"Add State(s) to Queue__JKI_lib_State_Machine.vi"("State(s) in Front (\"\")"="//Exit Sub-Modules ", "State(s) in (\"\")"=w382, "State(s) at Back (\"\")"="Data: Cleanup\nExit") -> ("States Out"=w384:string)  [unwired: 12 in]
                n115 = call <vilib>:"Add State(s) to Queue__JKI_lib_State_Machine.vi"("State(s) in Front (\"\")"=w384, "State(s) in (\"\")"=w389) -> ("States Out"=w388:string)  [unwired: 13 in]
              }
              frame "---------- API ----------" {
                # "#CSM \"Category Seperator\"\nDo not put any code in this frame."
              }
              frame "API: API1" {
                # "#CSM API Example\nCopy/Rename this case for your own API"
                # "#CSM Response\nConnect this to return the response of your API"
                # "#CSM >> Msg/Rep's CSM >>\nIf you need to tell who triggered this state , use this string. If it's this case itself, this string is \"\"."
                # "#CSM >> Arguments >>\nDeal with the parameter if any"
              }
              frame "API: API2" {
                # "#CSM API Example\nCopy/Rename this case for your own API"
                # "unpack Hex String  to Variant\nif complex parameter is needed."
                n116 = call "CSM - Convert HexStr to Data.vi"("HEX String"=w398) -> ()  [unwired: 7 in, 2 out]
                n117 = disable-structure shown="Disabled" {
                  disable-tunnel: [w402 "API2 Response"] -> w397
                  frame Disabled {
                    # "pack variant to hexstr \nif complex response is needed."
                    # "complex Response"
                    n118 = call "CSM - Convert Data to HexStr.vi"() -> ("HEX String (0-9,A-F)"=w402:string)  [unwired: 9 in]
                  }
                  frame Enabled {
                  }
                }
              }
              frame "---------- Action ----------" {
                # "#CSM \"Category Seperator\"\nDo not put any code in this frame."
                n119 = call <vilib>:"Add State(s) to Queue__JKI_lib_State_Machine.vi"("State(s) in (\"\")"=w407) -> ("States Out"=w406:string)  [unwired: 14 in]
              }
              frame "Action: action1" {
                # "#CSM \"Internal State\"\nThis category is used for holding internal states"
                n120 = call <vilib>:"Add State(s) to Queue__JKI_lib_State_Machine.vi"("State(s) in (\"\")"=w411) -> ("States Out"=w410:string)  [unwired: 14 in]
              }
              frame "Action: action2" {
                # "#CSM \"Internal State\"\nThis category is used for holding internal states"
                n121 = call <vilib>:"Add State(s) to Queue__JKI_lib_State_Machine.vi"("State(s) in (\"\")"=w415) -> ("States Out"=w414:string)  [unwired: 14 in]
              }
            }
          }
          n122 = for {
            shift-right: [w115] -> w85
            shift-left: w84 -> [w109]
            shift-right: [w121] -> w79
            shift-left: w89 -> [w110]
            tunnel: w88 -> [w130] mode=indexing
            i -> [w132]
            stop <- w115 stop-if-true
            w116 = "Handler Message" ("To")
            n123 = Unbundle By Name(w130) -> ("From"=w106:string, "To"=w105:string)
            n124 = Increment(x=w132) -> (x+1=→"LoopCount 2":i32)
            n125 = call "uuid.vi"() -> ("UUID"=w123:string)  [unwired: 11 in]
            n126 = Concatenate Strings(w106, " to " ("string"), w105) -> (w104:string)
            n127 = call "CSM - Wait and Send Message for Reply.vi"("State"="API: Test Register State", "Arguments (\"\")"=w123, "Target Module"=w106, "Error In (No Error)"=w109) -> ("error out"=w128:errorcluster)  [unwired: 8 in, 3 out]
            n128 = call "Stall Data Flow.vim"("value in"=w128, "milliseconds to wait"=u32 100) -> ("value out"=w126:errorcluster)  [unwired: 1 out]
            n129 = call "CSM Get Module Attribute.vim"("CSM Name"=w105, "Attribute"=w116, "Default Value (Empty Variant)"="", "Error In"=w126) -> ("CSM Name (Dup)"=w117:string, "Found"=w125:bool, "Value"=w122:string, "error out"=w118:errorcluster)  [unwired: 7 in, 1 out]
            n130 = flat-sequence {
              tunnel: w118 -> [w134]
              tunnel: w117 -> [w137]
              tunnel: w116 -> [w136]
              tunnel: [w133] -> w108
              frame #0 {
                n131 = call <vilib>:"Clear Errors.vi"("error in (no error)"=w134) -> ("error out"=w138:errorcluster)  [unwired: 5 in, 1 out]
                n132 = call "CSM - Delete Module Attribute.vi"("CSM Name"=w137, "Attribute"=w136, "Error In"=w138) -> ("error out"=w135:errorcluster)  [unwired: 9 in, 3 out]
                n133 = Merge Errors(w134, w135) -> (w133:errorcluster)
              }
            }
            n134 = call "Package Error Info.vi"("error in"=w108, "String in"=w104) -> ("packed error info out"=w113:string, "error status"=w114:bool)  [unwired: 8 in]
            n135 = Equal?(x=w123, y=w122) -> (x = y?=w120:bool)
            n136 = call-dynamic "failIf.vi"("message (\"\")"=w113, "fail"=w114, "TestCase in"=w110) -> ("error out"=w111:errorcluster, "TestCase out"=w112:refnum<class "testcase-CSMBroadcast.lvclass">)  [unwired: 7 in]
            n137 = And(x=w125, y=w120) -> (x .and. y?=w119:bool)
            n138 = call-dynamic "passIf.vi"("error in (no error)"=w111, "message (\"\")"=w104, "pass"=w119, "TestCase in"=w112) -> ("error out"=w115:errorcluster, "TestCase out"=w121:refnum<class "testcase-CSMBroadcast.lvclass">)  [unwired: 6 in]
          }
          n139 = flat-sequence {
            tunnel: w85 -> [w98]
            tunnel: [w97] -> w81
            tunnel: w79 -> [w96]
            tunnel: [w96] -> w78
            tunnel: w76 -> [w95]
            tunnel: w81 -> [w103]
            tunnel: [w102] -> w80
            tunnel: w78 -> [w100]
            tunnel: [w100] -> w77
            frame #0 {
              n140 = call "CSM - Send Message and Wait for Reply.vi"("Target Module"=w95, "State"="Macro: Exit") -> ("error out"=w94:errorcluster)  [unwired: 7 in, 2 out]
              n141 = call <vilib>:"Clear Errors.vi"("error in (no error)"=w94) -> ("error out"=w93:errorcluster)  [unwired: 5 in, 1 out]
              n142 = Merge Errors(w98, w93) -> (w97:errorcluster)
            }
            frame #1 {
              n143 = call "CSM - Drop Broadcast Registry.vi"() -> ("error out"=w101:errorcluster)  [unwired: 15 in]
              n144 = Merge Errors(w103, w101) -> (w102:errorcluster)
            }
          }
        }
      }
    }
    frame Disabled {
      # "skip test result while test is under development"
      n145 = call <vilib>:"skip.vi"("error in (no error)"=w416, "TestCase in"=w419) -> ("error out"=w418:errorcluster, "TestCase out"=w417:refnum<class "testcase-CSMBroadcast.lvclass">)  [unwired: 8 in]
    }
  }
  "error out" <- w4
  "TestCase out" <- w2
